vi "DLL_test.vi"() -> ()   [LabVIEW 2015]
doc: "This VI is used to test the funciton \"Call the Autofocus C++ dll\""
uses:
  focus_img.dll
  focus_array.dll
panel:
  out "Elapsed time (s)":dbl
  out "Finish time":dbl format="%_19f"
  out "Start time":dbl format="%_19f"
  in  "x":dbl[](array[numeric])=[1.0, 2.0, 3.0, 4.0]
  in  "Path 4":path=path "C:/Users/Administrator/Desktop/focus/3.png"
  in  "Path 3":path=path "C:/Users/Administrator/Desktop/focus/2.png"
  in  "Path 2":path=path "C:/Users/Administrator/Desktop/focus/1.png"
  out "BestPosition":dbl
  in  "Path":path=path "C:/Users/Administrator/Desktop/focus/0.png"
  # "This VI is used to test the funciton \"Call the Autofocus C++ dll\""
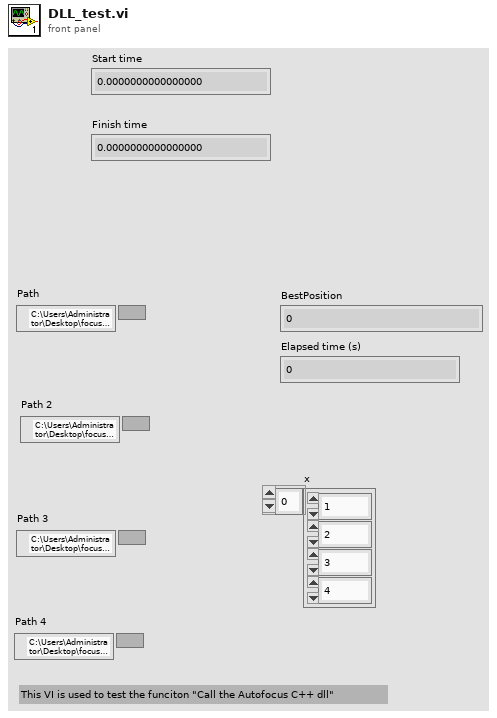
[diagram p1: front panel]
types:
  T1 = typedef "imagedata.ctl" = cluster{"image type":i32, "image depth":i32, "image":u8[], "mask":u8[], "colors":u32[], "Rectangle":cluster{"left":i16, "top":i16, "right":i16, "bottom":i16}}
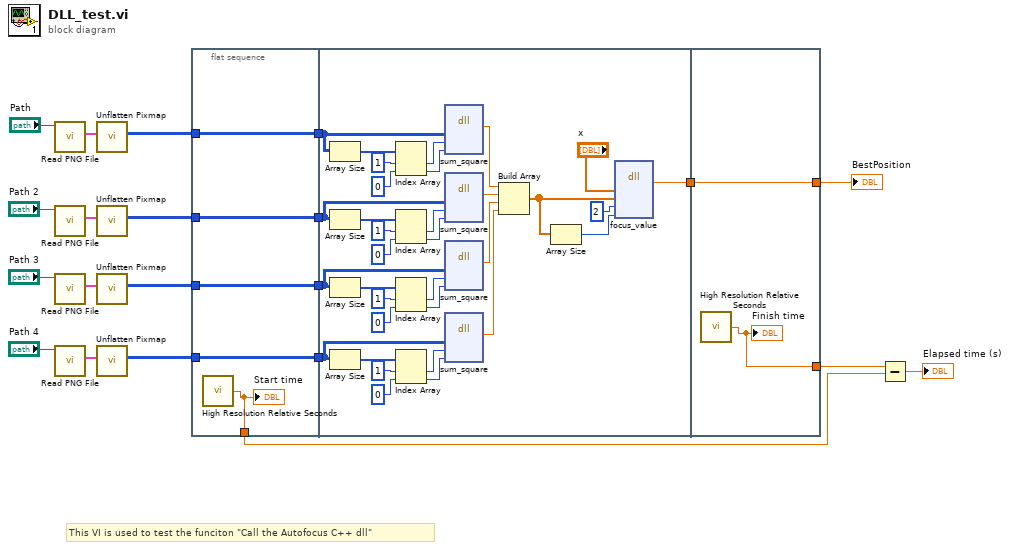
[diagram p0: block diagram]
diagram:
  # "This VI is used to test the funciton \"Call the Autofocus C++ dll\""
  n1 = call <vilib>:"Read PNG File.vi"("path to PNG file"="Path") -> ("image data"=w20:T1)  [unwired: 8 in, 2 out]
  n2 = call <vilib>:"Read PNG File.vi"("path to PNG file"="Path 2") -> ("image data"=w17:T1)  [unwired: 8 in, 2 out]
  n3 = call <vilib>:"Read PNG File.vi"("path to PNG file"="Path 3") -> ("image data"=w14:T1)  [unwired: 8 in, 2 out]
  n4 = call <vilib>:"Read PNG File.vi"("path to PNG file"="Path 4") -> ("image data"=w11:T1)  [unwired: 8 in, 2 out]
  n5 = call <vilib>:"Unflatten Pixmap.vi"("image data"=w20) -> ("8-bit pixmap"=w19:u8[][])  [unwired: 4 in, 6 out]
  n6 = call <vilib>:"Unflatten Pixmap.vi"("image data"=w17) -> ("8-bit pixmap"=w18:u8[][])  [unwired: 4 in, 6 out]
  n7 = call <vilib>:"Unflatten Pixmap.vi"("image data"=w14) -> ("8-bit pixmap"=w13:u8[][])  [unwired: 4 in, 6 out]
  n8 = call <vilib>:"Unflatten Pixmap.vi"("image data"=w11) -> ("8-bit pixmap"=w12:u8[][])  [unwired: 4 in, 6 out]
  n9 = flat-sequence {
    tunnel: w12 -> [w23]
    tunnel: w13 -> [w24]
    tunnel: w18 -> [w25]
    tunnel: w19 -> [w26]
    tunnel: [w26] -> w7
    tunnel: [w25] -> w6
    tunnel: [w24] -> w5
    tunnel: [w23] -> w4
    tunnel: [w22] -> w1
    tunnel: [w29] -> w8
    tunnel: w7 -> [w58]
    tunnel: w6 -> [w47]
    tunnel: w5 -> [w46]
    tunnel: w4 -> [w35]
    tunnel: [w61] -> w9
    tunnel: w8 -> [w61]
    tunnel: [w60] -> w2
    frame #0 {
      n10 = call <vilib>:"High Resolution Relative Seconds.vi"() -> ("relative seconds"=w22:dbl)
      "Start time" <- w22
    }
    frame #1 {
      n11 = Array Size(array=w58) -> (size(s)=w57:i32[])
      n12 = Array Size(array=w47) -> (size(s)=w48:i32[])
      n13 = Array Size(array=w46) -> (size(s)=w45:i32[])
      n14 = Array Size(array=w35) -> (size(s)=w36:i32[])
      n15 = Index Array(array=w57, index #1=1 ("index"), index #2=0 ("index")) -> (element #1=w54:i32, element #2=w53:i32)
      n16 = Index Array(array=w48, index #1=1 ("index"), index #2=0 ("index")) -> (element #1=w51:i32, element #2=w52:i32)
      n17 = Index Array(array=w45, index #1=1 ("index"), index #2=0 ("index")) -> (element #1=w42:i32, element #2=w41:i32)
      n18 = Index Array(array=w36, index #1=1 ("index"), index #2=0 ("index")) -> (element #1=w39:i32, element #2=w40:i32)
      n19 = dll-call lib="C:/Users/Administrator/Desktop/focus/DLL/DLL/focus_img.dll" fn="sum_square"("pBuffer"=w58, "width"=w54, "height"=w53) -> ("return type"=w59:dbl)  [unwired: 6 in, 2 out]
      n20 = dll-call lib="C:/Users/Administrator/Desktop/focus/DLL/DLL/focus_img.dll" fn="sum_square"("pBuffer"=w47, "width"=w51, "height"=w52) -> ("return type"=w34:dbl)  [unwired: 6 in, 2 out]
      n21 = dll-call lib="C:/Users/Administrator/Desktop/focus/DLL/DLL/focus_img.dll" fn="sum_square"("pBuffer"=w46, "width"=w42, "height"=w41) -> ("return type"=w33:dbl)  [unwired: 6 in, 2 out]
      n22 = dll-call lib="C:/Users/Administrator/Desktop/focus/DLL/DLL/focus_img.dll" fn="sum_square"("pBuffer"=w35, "width"=w39, "height"=w40) -> ("return type"=w32:dbl)  [unwired: 6 in, 2 out]
      n23 = Build Array(w59, w34, w33, w32) -> (w28:dbl[])
      n24 = Array Size(array=w28) -> (size(s)=w27:i32)
      n25 = dll-call lib="C:/Users/Administrator/Desktop/focus/DLL/DLL/focus_array.dll" fn="focus_value"("x"="x", "y"=w28, "pow"=2, "total"=w27) -> ("return type"=w29:dbl)  [unwired: 7 in, 2 out]
    }
    frame #2 {
      n26 = call <vilib>:"High Resolution Relative Seconds.vi"() -> ("relative seconds"=w60:dbl)
      "Finish time" <- w60
    }
  }
  n27 = Subtract(x=w2, y=w1) -> (x-y=→"Elapsed time (s)":dbl)
  "BestPosition" <- w9
